vi "DriveForDistance-C.vi"(11 "Params":string[][](array[string])) -> ()   [LabVIEW 2017]
uses:
  C:/Users/competition/Documents/LabVIEW Data/Projects/FRC_PracticeBot-2018/Robot Project/Framework/Robot Global Data.vi
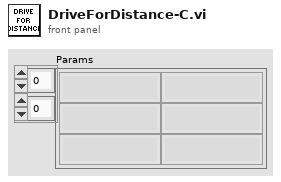
[diagram p1: front panel]
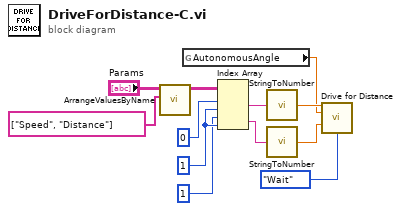
[diagram p0: block diagram]
diagram:
  w5 = 1
  n1 = call "ArrangeValuesByName.vi"("Names"=string[] ["Speed", "Distance"], "Names/Values in"="Params") -> ("Names/Values Out"=w7:string[][])  [unwired: 9 in]
  n2 = global read "Robot Global Data.vi" "AutonomousAngle"() -> (w10:dbl)
  n3 = Index Array(array=w7, index (row) #1=0, index (col) #1=w5, index (row) #2=1, index (col) #2=w5) -> (element #1=w3:string, element #2=w1:string)
  n4 = call "StringToNumber.vi"("String"=w3) -> ("Output"=w12:dbl)
  n5 = call "StringToNumber.vi"("String"=w1) -> ("Output"=w11:dbl)
  n6 = call "Drive for Distance.vi"("Speed"=w12, "StartAngle"=w10, "Distance (inch)"=w11, "Synchronication"=enum16{"Start", "Wait"}."Wait") -> ()  [unwired: 11 in, 1 out]
